vi "Image.vi"(2 "XRef":refnum<vi>, 3 "State In":T1={"Input Type"=variant(dbl 0.0), "Selection"=0, "Element Names"=[], "Type Strings"=[], "Element Types"=[]}) -> (0 "Image":picture)   [LabVIEW 2015, in "Case-Tagged-Union.xnode"]
doc: "This ability VI is used to describe your XNode's appearance. The origin of Image corresponds to the top-left corner of your XNode. The bounds of your XNode are used to crop this image. If you want LabVIEW to update your image, you need to inform it through the UpdateImage or UpdateImageAndBounds replies. Any areas where you do not draw are transparent, so regions intended to appear white should be explicitly drawn.\n \n Remember to localize any strings that are part of your image.\n\nDefault behavior: None.\n\nThis ability does not provide UI and OS messages are not handled."
uses:
  Case-Tagged-Union.xnode
  State.ctl
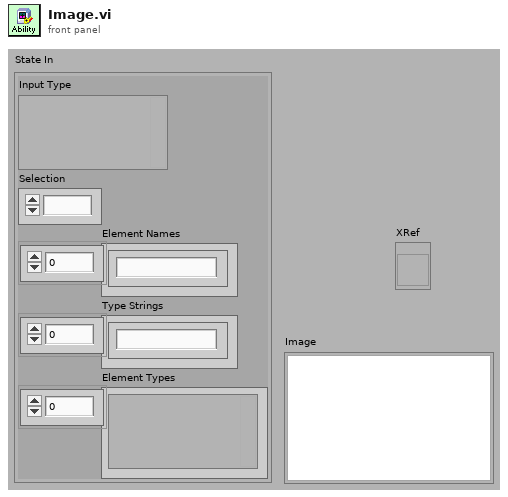
[diagram p1: front panel]
types:
  T1 = typedef "Case-Tagged-Union.xnode/State.ctl" = cluster{"Input Type":variant, "Selection":i32, "Element Names":string[], "Type Strings":string[], "Element Types":variant[]}
  T2 = typedef "imagedata.ctl" = cluster{"image type":i32, "image depth":i32, "image":u8[], "mask":u8[], "colors":u32[], "Rectangle":cluster{"left":i16, "top":i16, "right":i16, "bottom":i16}}
  T3 = cluster{"left":i16, "top":i16, "right":i16, "bottom":i16}
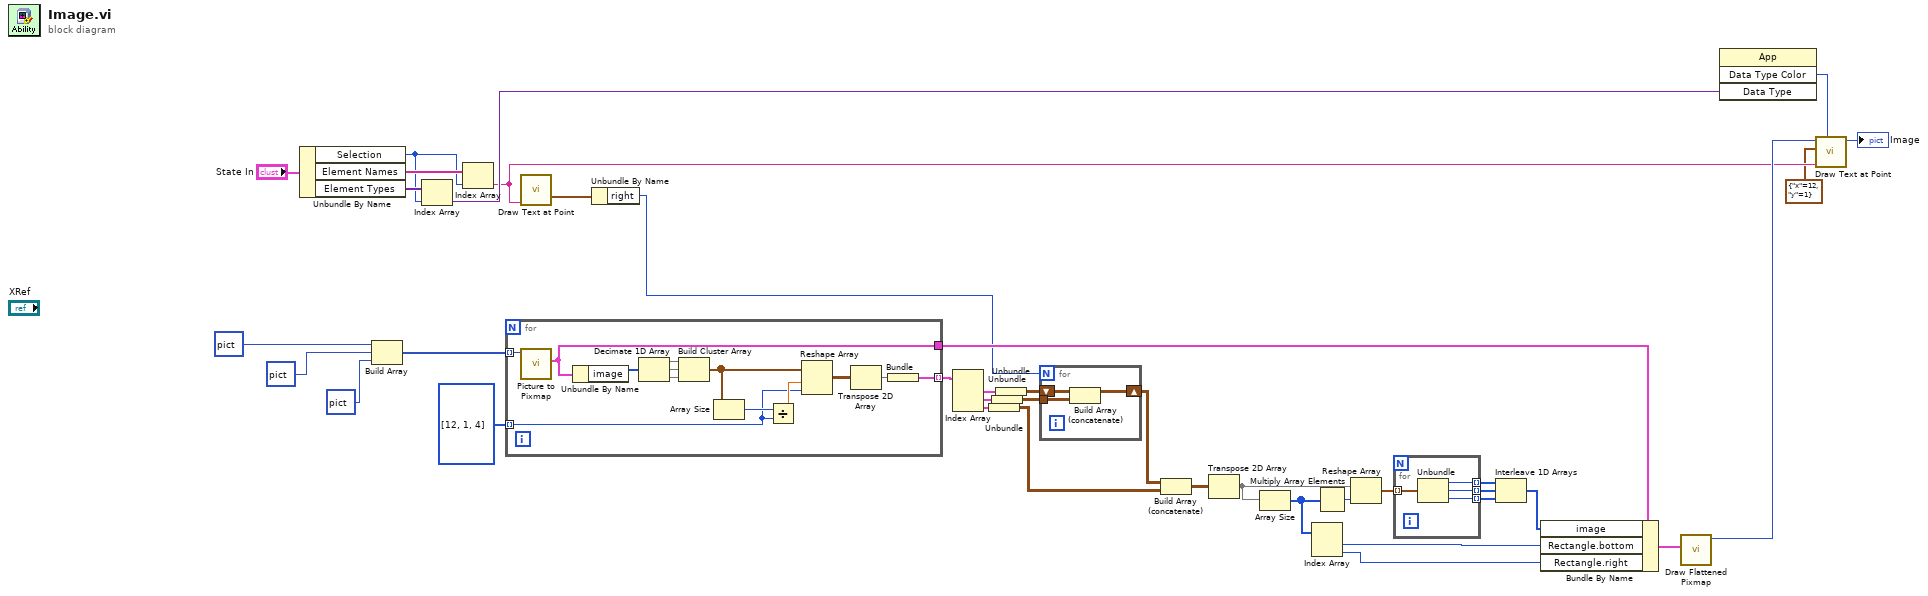
[diagram p0: block diagram]
diagram:
  n1 = Unbundle By Name("State In") -> ("Selection"=w33:i32, "Element Names"=w34:string[], "Element Types"=w35:variant[])
  n2 = Build Array(picture bytes[752] ("new picture"), picture bytes[87] ("new picture"), picture bytes[296] ("new picture")) -> (w11:picture[])
  n3 = Index Array(array=w35, index=w33) -> (element=w9:variant)
  n4 = Index Array(array=w34, index=w33) -> (element=w8:string)
  n5 = for {
    tunnel: w11 -> [w51] mode=indexing
    tunnel: i32[] [12, 1, 4] -> [w43] mode=indexing
    tunnel: [w40] -> w31 mode=indexing
    tunnel: [w39] -> w16
    n6 = call <vilib>:"Picture to Pixmap.vi"("picture"=w51) -> ("image data"=w39:T2)  [unwired: 9 in, 1 out]
    n7 = Unbundle By Name(w39) -> ("image"=w47:u8[])
    n8 = Decimate 1D Array(w47) -> (w46:u8[], w44:u8[], w45:u8[])
    n9 = Build Cluster Array(w46, w44, w45) -> (w48:cluster{u8, u8, u8}[])
    n10 = Array Size(array=w48) -> (size(s)=w49:i32)
    n11 = Divide(x=w49, y=w43) -> (x/y=w50:dbl)
    n12 = Reshape Array(w48, w50, w43) -> (w42:cluster{u8, u8, u8}[][])
    n13 = Transpose 2D Array(2D array=w42) -> (transposed array=w41:cluster{u8, u8, u8}[][])
    n14 = Bundle(w41) -> (w40:cluster{cluster{u8, u8, u8}[][]})  [unwired: 1 in]
  }
  n15 = call <vilib>:"Draw Text at Point.vi"("text"=w8) -> ("text rect"=w7:T3)  [unwired: 9 in, 1 out]
  n16 = Unbundle By Name(w7) -> ("right"=w6:i16)
  n17 = Index Array(array=w31) -> (element #1=w29:cluster{cluster{u8, u8, u8}[][]}, element #2=w30:cluster{cluster{u8, u8, u8}[][]}, element #3=w27:cluster{cluster{u8, u8, u8}[][]})  [unwired: 3 in]
  n18 = Unbundle(w27) -> (w12:cluster{u8, u8, u8}[][])
  n19 = Unbundle(w30) -> (w13:cluster{u8, u8, u8}[][])
  n20 = Unbundle(w29) -> (w14:cluster{u8, u8, u8}[][])
  n21 = for {
    N: w6 -> [_]
    shift-right: [w52] -> w28
    shift-left: w14 -> [w53]
    tunnel: w13 -> [w54]
    n22 = Build Array (concatenate)(w53, w54) -> (w52:cluster{u8, u8, u8}[][])
  }
  n23 = Build Array (concatenate)(w28, w12) -> (w26:cluster{u8, u8, u8}[][])
  n24 = Transpose 2D Array(2D array=w26) -> (transposed array=w17:cluster{u8, u8, u8}[][])
  n25 = Array Size(array=w17) -> (size(s)=w25:i32[])
  n26 = Index Array(array=w25) -> (element #1=w18:i32, element #2=w15:i32)  [unwired: 2 in]
  n27 = Multiply Array Elements(1:w25) -> (0:w24:i32)
  n28 = Reshape Array(w17, w24) -> (w23:cluster{u8, u8, u8}[])
  n29 = for {
    tunnel: w23 -> [w58] mode=indexing
    tunnel: [w57] -> w22 mode=indexing
    tunnel: [w56] -> w21 mode=indexing
    tunnel: [w55] -> w20 mode=indexing
    n30 = Unbundle(w58) -> (w57:u8, w56:u8, w55:u8)
  }
  n31 = Interleave 1D Arrays(w22, w21, w20) -> (w19:u8[])
  n32 = Bundle By Name(cluster=w16, "image"=w19, "Rectangle.bottom"=w18, "Rectangle.right"=w15) -> (w10:T2)
  n33 = call <vilib>:"Draw Flattened Pixmap.vi"("image data"=w10) -> ("new picture"=w37:picture)  [unwired: 1 in, 7 out]
  n34 = invoke class="App" method="Data Type Color"("Data Type"=w9) -> ("Data Type Color"=w36:u32)  [unwired: 3 in, 3 out]
  n35 = call <vilib>:"Draw Text at Point.vi"("text color(black)"=w36, "text"=w8, "origin"=cluster{"x":i16, "y":i16} {"x"=12, "y"=1}, "picture"=w37) -> ("new picture"=→"Image":picture)  [unwired: 6 in, 1 out]
